vi "Agilent 3458 Acquire Multiple Measurement.vi"(0 "VISA resource name":refnum<visa-resource-name>, 1 "Function (0: DC Voltage)":u16(ring) items=["DC Voltage", "AC Voltage", "AC + DC Voltage", "DC Current", "AC Current", "AC + DC Current", "2-Wire Resistance", "4-Wire Resistance", "Frequency", "Period", "Direct Sampling DC", "Direct Sampling AC"], 2 "Sample Count (1)":dbl=10.0 format="%#.6g", 3 "Trigger Count (1)":dbl=1.0, 4 "Init":bool, 5 "Reset":bool, 7 "Manual Resolution (2: 6.5 digits)":enum16{"4.5", "5.5", "6.5", "7.5", "8.5"}(ring)=enum."6.5", 9 "Integration Time (0 PLCs)":dbl, 11 "error in (no error)":errorcluster, 12 "Auto Range (1:ON)":u16(ring)=1 items=["OFF", "ON", "ONCE"], 13 "Maximum Time (10000 ms)":u32=10000, 14 "Manual Range (1.00)":dbl=1.0 format="%_3g") -> (6 "Measurements":sgl[](array[numeric]), 15 "error out":errorcluster)   [LabVIEW 2016]
doc: "Shows how to configure a measurement and take multiple readings."
uses:
  <userlib>/_TI-LA/Instr Drivers/Multimeter/E3458/Driver/Base/Public/Data/Read Measurement(Multiple Points).vi
  <userlib>/_TI-LA/Instr Drivers/Multimeter/E3458/Driver/E3458.lvlib
panel:
  in  "Frequency Source (3: AC Voltage)":u16(ring)=3 items=["AC + DC Current", "AC + DC Voltage", "AC Current", "AC Voltage"]
  in  "Trigger Type (0:Auto)":u16(ring) items=["Auto", "External", "Level", "Line", "Synchronous"]
  # "(c) 2007  National Instruments.  ALL RIGHTS RESERVED."
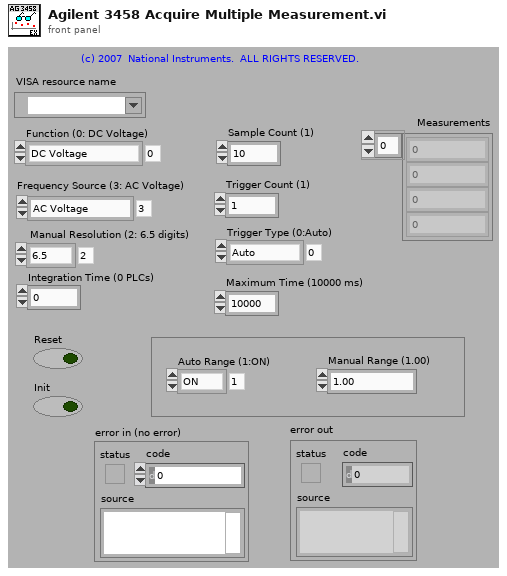
[diagram p1: front panel]
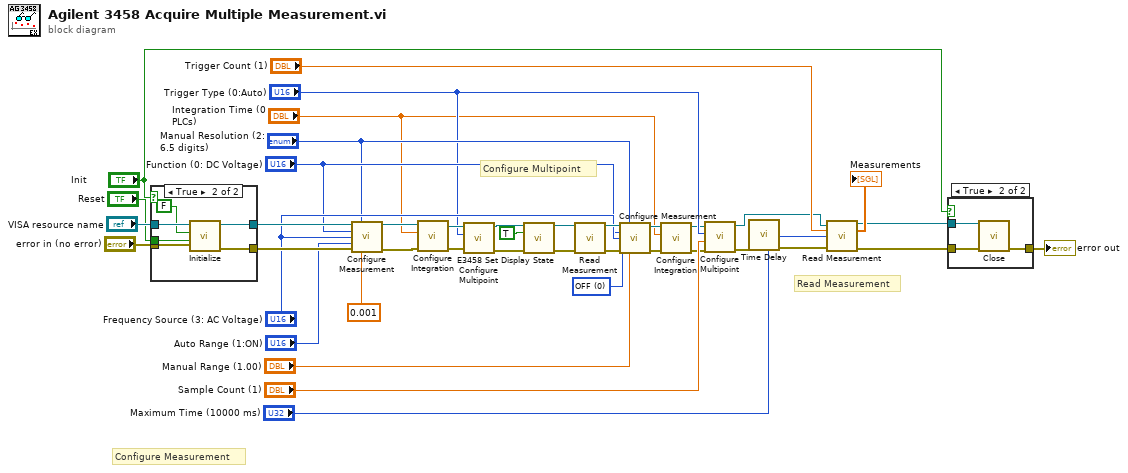
[diagram p0: block diagram]
diagram:
  w15 = u16 0 items=["OFF", "ON", "ONCE"] ("Auto Range (1:ON)")
  # "Configure Multipoint"
  # "Read Measurement"
  # "Configure Measurement"
  n1 = case shown="True" "Init" {
    tunnel: "VISA resource name" -> [w42 w48]
    tunnel: [w42 w47] -> w37
    tunnel: [w41 w46] -> w36
    tunnel: "error in (no error)" -> [w41 w45]
    tunnel: "Reset" -> [_ w44]
    frame False {
    }
    frame True {
      n2 = call <userlib>:"Initialize.vi"("error in (no error)"=w45, "Reset (True)"=w44, "ID Query (True)"=FALSE, "VISA resource name"=w48) -> ("error out"=w46:errorcluster, "VISA resource name out"=w47:refnum<visa-resource-name>)  [unwired: 1 in, 5 out]
    }
  }
  n3 = call <userlib>:"Configure Measurement.vi"("VISA resource name"=w37, "Manual Resolution (2: 6.5 digits)"="Manual Resolution (2: 6.5 digits)", "Function (0: DC Voltage)"="Function (0: DC Voltage)", "Frequency Source (3: AC Voltage)"="Frequency Source (3: AC Voltage)", "Auto Range (1:ON)"="Auto Range (1:ON)", "error in (no error)"=w36, "Manual Range (1.00)"=0.001) -> ("VISA resource name out"=w30:refnum<visa-resource-name>, "error out"=w29:errorcluster)  [unwired: 1 in, 6 out]
  n4 = call <userlib>:"Configure Integration.vi"("error in (no error)"=w29, "Integration Time (0 PLCs)"="Integration Time (0 PLCs)", "VISA resource name"=w30) -> ("error out"=w28:errorcluster, "VISA resource name out"=w27:refnum<visa-resource-name>)  [unwired: 7 in]
  n5 = call <userlib>:"Configure Multipoint.vi"("error in (no error)"=w28, "Trigger Type (0:Auto)"="Trigger Type (0:Auto)", "VISA resource name"=w27) -> ("error out"=w24:errorcluster, "VISA resource name out"=w25:refnum<visa-resource-name>)  [unwired: 1 in, 6 out]
  n6 = call <userlib>:"E3458 Set Display State.vi"("VISA resource name"=w25, "Display State?"=TRUE, "error in"=w24) -> ("VISA resource name out"=w19:refnum<visa-resource-name>, "error out"=w18:errorcluster)  [unwired: 11 in]
  n7 = call-poly <userlib>:"Read Measurement.vi"("VISA resource name"=w19, "error in (no error)"=w18) -> ("VISA resource name out"=w17:refnum<visa-resource-name>, "error out"=w16:errorcluster)  [unwired: 2 in, 10 out]
  n8 = call <userlib>:"Configure Measurement.vi"("VISA resource name"=w17, "Manual Resolution (2: 6.5 digits)"="Manual Resolution (2: 6.5 digits)", "Function (0: DC Voltage)"="Function (0: DC Voltage)", "Frequency Source (3: AC Voltage)"="Frequency Source (3: AC Voltage)", "Auto Range (1:ON)"=w15, "error in (no error)"=w16, "Manual Range (1.00)"="Manual Range (1.00)") -> ("VISA resource name out"=w4:refnum<visa-resource-name>, "error out"=w5:errorcluster)  [unwired: 1 in, 6 out]
  n9 = call <userlib>:"Configure Integration.vi"("error in (no error)"=w5, "Integration Time (0 PLCs)"="Integration Time (0 PLCs)", "VISA resource name"=w4) -> ("error out"=w1:errorcluster, "VISA resource name out"=w2:refnum<visa-resource-name>)  [unwired: 7 in]
  n10 = call <userlib>:"Configure Multipoint.vi"("error in (no error)"=w1, "Sample Count (1)"="Sample Count (1)", "Trigger Type (0:Auto)"="Trigger Type (0:Auto)", "VISA resource name"=w2) -> ("error out"=w6:errorcluster, "VISA resource name out"=w7:refnum<visa-resource-name>)  [unwired: 6 out]
  n11 = call "Time Delay"("error in (no error)"=w6) -> ("error out"=w22:errorcluster)  [unwired: 10 in]
  n12 = call-poly <userlib>:"Read Measurement.vi"("VISA resource name"=w7, "Trigger Count (1)"="Trigger Count (1)", "Maximum Time (10000 ms)"="Maximum Time (10000 ms)", "error in (no error)"=w22) -> ("VISA resource name out"=w35:refnum<visa-resource-name>, "Measurements"=→"Measurements":sgl[], "error out"=w34:errorcluster)  [unwired: 9 out]
  n13 = case shown="True" "Init" {
    tunnel: [w49 w52] -> w40
    tunnel: w35 -> [_ w51]
    tunnel: w34 -> [w49 w50]
    frame False {
    }
    frame True {
      n14 = call <userlib>:"Close.vi"("error in (no error)"=w50, "VISA resource name"=w51) -> ("error out"=w52:errorcluster)  [unwired: 9 out]
    }
  }
  "error out" <- w40
